vi "ReadResizePanel__slk_mt.vi"(8 "error in (no error)":errorcluster, 11 "refnum in":T1) -> (0 "error out":errorcluster, 2 "resize panel configure":T2={"Set Front Panel"=FALSE, "FP Frame Width"=0, "FP Position"="Top Left", "Set Origin"=FALSE, "Ignore Hidden"=FALSE, "Ignore Decorations"=FALSE, "Set Block Diagram"=FALSE, "BD Frame Width"=0}, 3 "refnum out":T1)   [LabVIEW 2010, in "Lazyboots Menu Tool.lvlib"]
doc: "Gets configure datum of Resize Panel.\n\n<b>[Resize Panel]</b>\nSet Front Panel = \"TRUE\"\nFP Frame Width = \"20\"\nFP Position = \"Top Left\"\nSet Origin = \"TRUE\"\nIgnore Hidden = \"TRUE\"\nIgnore Decorations = \"FALSE\"\nSet Block Diagram = \"TRUE\"\nBD Frame Width = \"20\""
uses:
  Library/Lazyboots Menu Tool.lvlib
  TypeDef/TypeDef_ResizePanelConfigure__slk_mt.ctl
  <vilib>/Utility/config.llb/Config Data RefNum.ctl
  <vilib>/Utility/config.llb/Read Key (Boolean).vi
  <vilib>/Utility/config.llb/Read Key (U32).vi
  <vilib>/Utility/config.llb/Read Key (String).vi
  <vilib>/Utility/config.llb/NI_LVConfig.lvlib
panel:
  # "ReadResizePanel__slk_mt.vi\nGets configure datum of Resize Panel.\n\nNOTICE -- YOU MUST LEAVE THIS NOTICE IN PLACE.\n\nCopyright (c) 2011, LIANG LIU Shawn.Liu.cn@gmail.com\nAll rights reserved.\n\nRedistribution and use in source and binary forms, with or without modification, are permitted provided that the following conditions are met:\n-Redistributions of source code must retain the above copyright notice, this list of conditions and the following disclaimer.\n-Redistributions in binary form must reproduce the above copyright notice, this list of conditions and the following disclaimer in the documentation and/or other materials provided with the distribution.\n-Neither the name of the eLp nor the names of its contributors may be used to endorse or promote products derived from this software without specific prior written permission.\n\nTHIS SOFTWARE IS PROVIDED BY THE COPYRIGHT HOLDERS AND CONTRIBUTORS \"AS IS\" AND ANY EXPRESS OR IMPLIED WARRANTIES, INCLUDING, BUT NOT LIMITED TO, THE IMPLIED WARRANTIES OF MERCHANTABILITY AND FITNESS FOR A PARTICULAR PURPOSE ARE DISCLAIMED. IN NO EVENT SHALL THE COPYRIGHT HOLDER OR CONTRIBUTORS BE LIABLE FOR ANY DIRECT, INDIRECT, INCIDENTAL, SPECIAL, EXEMPLARY, OR CONSEQUENTIAL DAMAGES (INCLUDING, BUT NOT LIMITED TO, PROCUREMENT OF SUBSTITUTE GOODS OR SERVICES; LOSS OF USE, DATA, OR PROFITS; OR BUSINESS INTERRUPTION) HOWEVER CAUSED AND ON ANY THEORY OF LIABILITY, WHETHER IN CONTRACT, STRICT LIABILITY, OR TORT (INCLUDING NEGLIGENCE OR OTHERWISE) ARISING IN ANY WAY OUT OF THE USE OF THIS SOFTWARE, EVEN IF ADVISED OF THE POSSIBILITY OF SUCH DAMAGE."
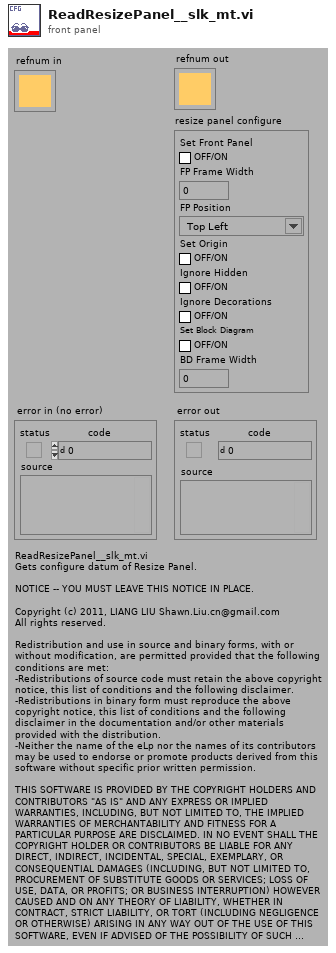
[diagram p1: front panel]
types:
  T1 = typedef "NI_LVConfig.lvlib/Config Data RefNum.ctl" = refnum<k1>
  T2 = typedef "Lazyboots Menu Tool.lvlib/TypeDef_ResizePanelConfigure__slk_mt.ctl" = cluster{"Set Front Panel":bool, "FP Frame Width":u32, "FP Position":string, "Set Origin":bool, "Ignore Hidden":bool, "Ignore Decorations":bool, "Set Block Diagram":bool, "BD Frame Width":u32}
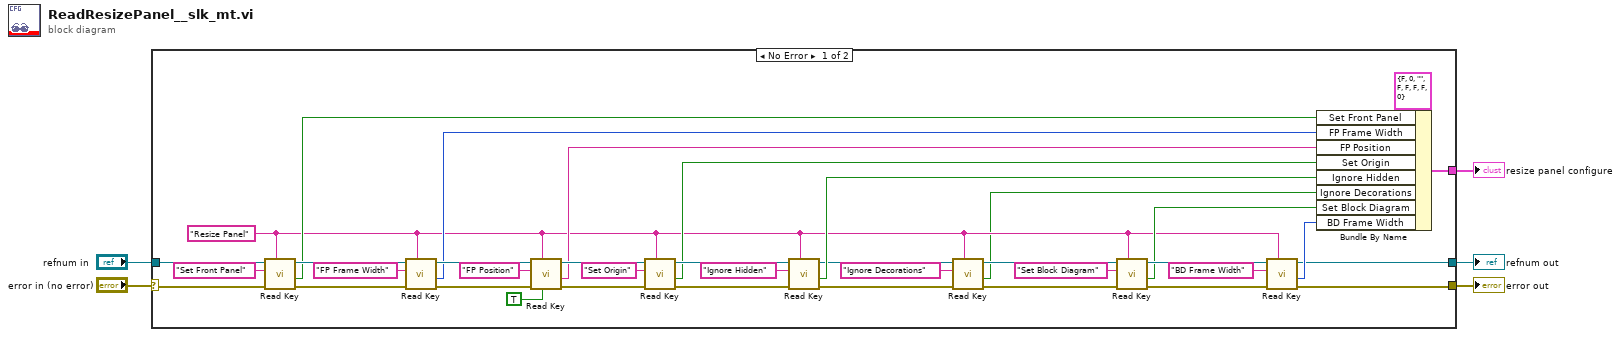
[diagram p0: block diagram]
diagram:
  n1 = case shown="No Error" "error in (no error)" {
    selector: "error in (no error)" -> [w21 w45]
    tunnel: "refnum in" -> [w24 w44]
    tunnel: [w7 w44] -> w4
    tunnel: [w40 _] -> w2
    tunnel: [w6 w45] -> w1
    frame No Error {
      w12 = "Resize Panel" ("section")
      n2 = call-poly <vilib>:"Read Key.vi"("section"=w12, "error in (no error)"=w21, "key"="Set Front Panel", "refnum"=w24) -> ("error out"=w23:errorcluster, "value"=w19:bool, "refnum out"=w22:T1)  [unwired: 4 in, 1 out]
      n3 = call-poly <vilib>:"Read Key.vi"("section"=w12, "error in (no error)"=w23, "key"="FP Frame Width", "refnum"=w22) -> ("error out"=w36:errorcluster, "value"=w41:u32, "refnum out"=w43:T1)  [unwired: 4 in, 1 out]
      n4 = call-poly <vilib>:"Read Key.vi"("read raw string? (F)"=TRUE, "section"=w12, "error in (no error)"=w36, "key"="FP Position", "refnum"=w43) -> ("error out"=w35:errorcluster, "value"=w34:string, "refnum out"=w37:T1)  [unwired: 3 in, 1 out]
      n5 = call-poly <vilib>:"Read Key.vi"("section"=w12, "error in (no error)"=w35, "key"="Set Origin", "refnum"=w37) -> ("error out"=w31:errorcluster, "value"=w29:bool, "refnum out"=w32:T1)  [unwired: 4 in, 1 out]
      n6 = call-poly <vilib>:"Read Key.vi"("section"=w12, "error in (no error)"=w31, "key"="Ignore Hidden", "refnum"=w32) -> ("error out"=w14:errorcluster, "value"=w30:bool, "refnum out"=w10:T1)  [unwired: 4 in, 1 out]
      n7 = call-poly <vilib>:"Read Key.vi"("section"=w12, "error in (no error)"=w14, "key"="Ignore Decorations", "refnum"=w10) -> ("error out"=w13:errorcluster, "value"=w9:bool, "refnum out"=w11:T1)  [unwired: 4 in, 1 out]
      n8 = call-poly <vilib>:"Read Key.vi"("section"=w12, "error in (no error)"=w13, "key"="Set Block Diagram", "refnum"=w11) -> ("error out"=w16:errorcluster, "value"=w15:bool, "refnum out"=w17:T1)  [unwired: 4 in, 1 out]
      n9 = call-poly <vilib>:"Read Key.vi"("section"=w12, "error in (no error)"=w16, "key"="BD Frame Width", "refnum"=w17) -> ("error out"=w6:errorcluster, "value"=w25:u32, "refnum out"=w7:T1)  [unwired: 4 in, 1 out]
      n10 = Bundle By Name(cluster=T2 {"Set Front Panel"=FALSE, "FP Frame Width"=0, "FP Position"="", "Set Origin"=FALSE, "Ignore Hidden"=FALSE, "Ignore Decorations"=FALSE, "Set Block Diagram"=FALSE, "BD Frame Width"=0} ("Resize Panel Configure"), "Set Front Panel"=w19, "FP Frame Width"=w41, "FP Position"=w34, "Set Origin"=w29, "Ignore Hidden"=w30, "Ignore Decorations"=w9, "Set Block Diagram"=w15, "BD Frame Width"=w25) -> (w40:T2)
    }
    frame Error {
    }
  }
  "resize panel configure" <- w2
  "error out" <- w1
  "refnum out" <- w4
